vi "FGV_MainPanel.vi"(8 "error in":errorcluster, 10 "LS_U8":u8, 11 "Estado":T2) -> (0 "error out":errorcluster, 2 "Finales_Carrera_Valores":T1)   [LabVIEW 2026]
uses:
  Cluster_ValorFinalesCarrera.ctl
  Ctrl_MainPanelGui.ctl
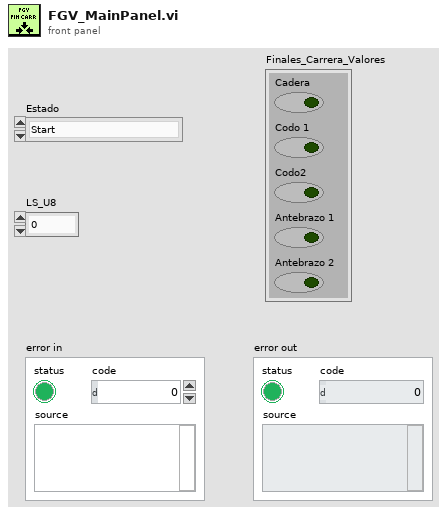
[diagram p1: front panel]
types:
  T1 = typedef "Cluster_ValorFinalesCarrera.ctl" = cluster{"Cadera":bool, "Codo 1":bool, "Codo2":bool, "Antebrazo 1":bool, "Antebrazo 2":bool}
  T2 = typedef "Ctrl_MainPanelGui.ctl" = enum16{"Start", "SET_DATA", "GET_DATA", "STOP"}
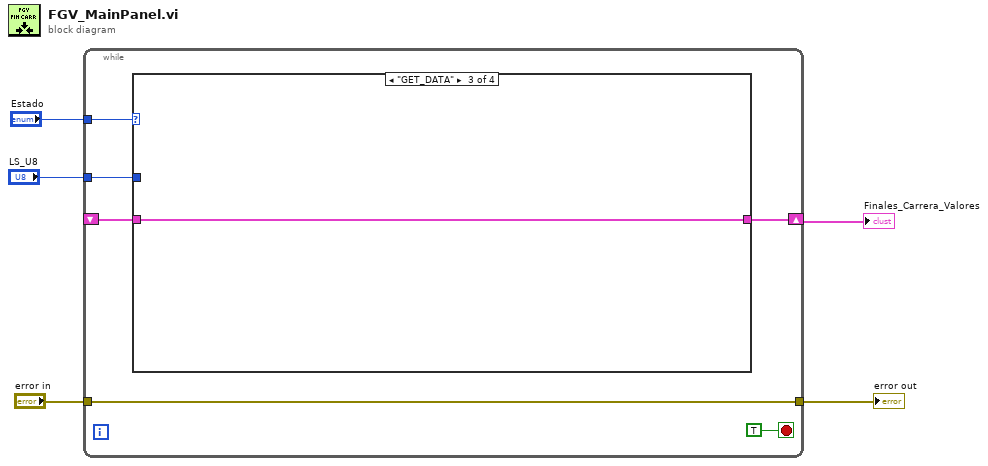
[diagram p0: block diagram]
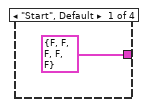
[diagram p2: hidden frame]
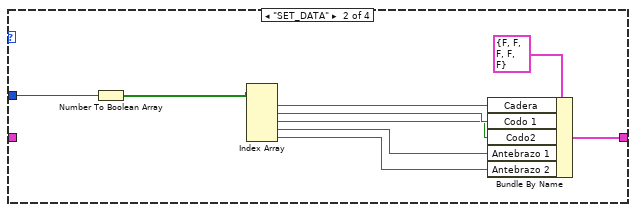
[diagram p3: hidden frame]
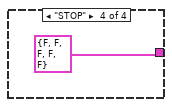
[diagram p4: hidden frame]
diagram:
  n1 = while {
    tunnel: "error in" -> [w10]
    tunnel: [w10] -> w4
    tunnel: "Estado" -> [w9]
    shift-right: [w8] -> w2
    shift-left: _ -> [w6]
    tunnel: "LS_U8" -> [w7]
    stop <- TRUE stop-if-true
    n2 = case shown="\"GET_DATA\"" w9 {
      tunnel: [T1 {"Cadera"=FALSE, "Codo 1"=FALSE, "Codo2"=FALSE, "Antebrazo 1"=FALSE, "Antebrazo 2"=FALSE} w20 w22 T1 {"Cadera"=FALSE, "Codo 1"=FALSE, "Codo2"=FALSE, "Antebrazo 1"=FALSE, "Antebrazo 2"=FALSE}] -> w8
      tunnel: w7 -> [_ w21 _ _]
      tunnel: w6 -> [_ _ w22 _]
      frame "Start", Default {
      }
      frame "SET_DATA" {
        n3 = Number To Boolean Array(number=w21) -> (Boolean array=w18:bool[])
        n4 = Index Array(array=w18) -> (element #1=w17:bool, element #2=w16:bool, element #3=w15:bool, element #4=w14:bool, element #5=w13:bool)  [unwired: 5 in]
        n5 = Bundle By Name(cluster=T1 {"Cadera"=FALSE, "Codo 1"=FALSE, "Codo2"=FALSE, "Antebrazo 1"=FALSE, "Antebrazo 2"=FALSE}, "Cadera"=w17, "Codo 1"=w16, "Codo2"=w15, "Antebrazo 1"=w14, "Antebrazo 2"=w13) -> (w20:T1)
      }
      frame "GET_DATA" {
      }
      frame "STOP" {
      }
    }
  }
  "error out" <- w4
  "Finales_Carrera_Valores" <- w2
